vi "VI Leer.vi"   [LabVIEW 2020]
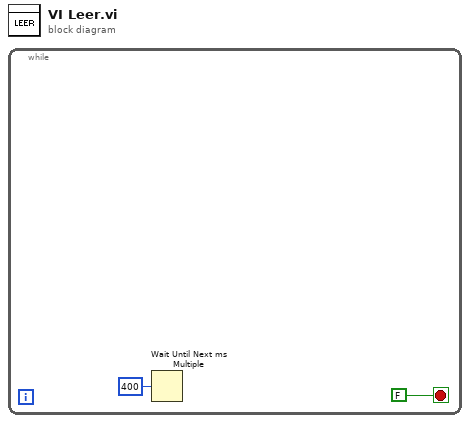
[diagram p0: block diagram]
diagram:
  n1 = while {
    stop <- FALSE stop-if-true
    n2 = Wait Until Next ms Multiple(millisecond multiple=u32 400 ("Zu wartende ms")) -> ()  [unwired: 1 out]
  }
